vi "Read Network-published IO Shared Variables.vi"() -> (1 "channel errors":errorcluster[](array[cluster]), 2 "data":dbl[](array[numeric]), 3 "UUIDs":string[](array[string])=["Flow Rate [g/s]", "Density [g/cm^3]", "Return Filter dP [psid]", "Outlet Filter and Flowmeter dp [psid]", "Cooler dP [psid]", "Cooler CO2 In [F]", "Cooler CO2 Out [F]", "Pump Frequency [%]", "Recirc Valve Open [%]"])   [LabVIEW 2020]
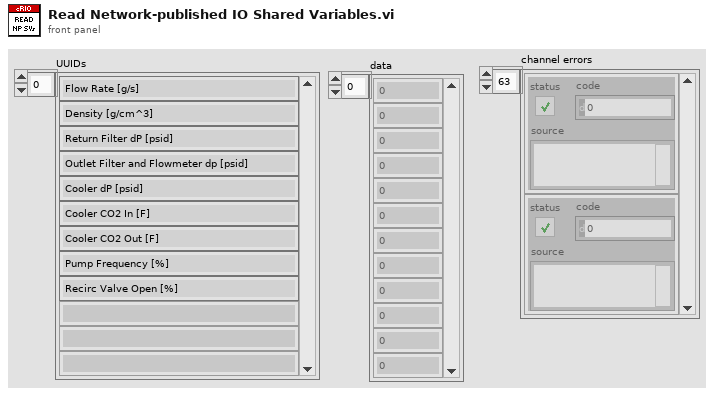
[diagram p1: front panel]
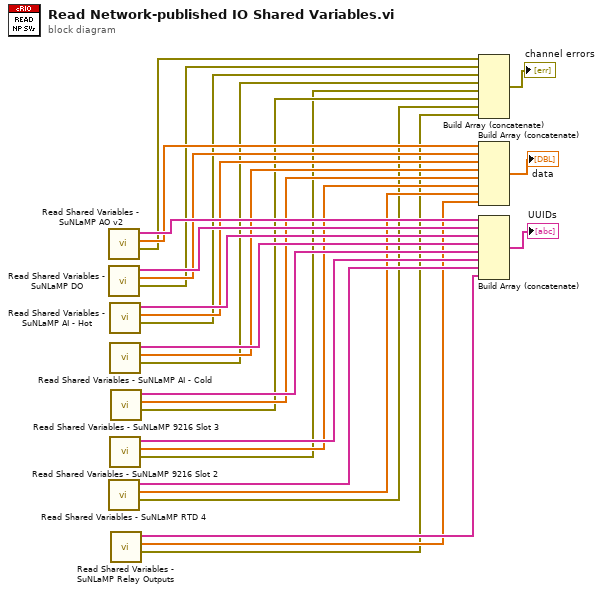
[diagram p0: block diagram]
diagram:
  n1 = call "Read Shared Variables - SuNLaMP AO v2.vi"() -> ("channel errors out"=w16:errorcluster[], "data"=w20:dbl[], "UUIDs"=w27:string[])  [unwired: 9 in]
  n2 = call "Read Shared Variables - SuNLaMP DO.vi"() -> ("channel errors out"=w17:errorcluster[], "data"=w21:dbl[], "UUIDs"=w26:string[])  [unwired: 9 in]
  n3 = call "Read Shared Variables - SuNLaMP RTD 4.vi"() -> ("channel errors out"=w4:errorcluster[], "data"=w5:dbl[], "UUIDs"=w6:string[])  [unwired: 9 in]
  n4 = call "Read Shared Variables - SuNLaMP AI - Hot.vi"() -> ("channel errors out"=w18:errorcluster[], "data"=w22:dbl[], "UUIDs"=w25:string[])  [unwired: 9 in]
  n5 = call "Read Shared Variables - SuNLaMP AI - Cold.vi"() -> ("channel errors out"=w19:errorcluster[], "data"=w23:dbl[], "UUIDs"=w24:string[])  [unwired: 9 in]
  n6 = call "Read Shared Variables - SuNLaMP 9216 Slot 2.vi"() -> ("channel errors out"=w7:errorcluster[], "data"=w8:dbl[], "UUIDs"=w11:string[])  [unwired: 9 in]
  n7 = call "Read Shared Variables - SuNLaMP 9216 Slot 3.vi"() -> ("channel errors out"=w9:errorcluster[], "data"=w10:dbl[], "UUIDs"=w12:string[])  [unwired: 9 in]
  n8 = call "Read Shared Variables - SuNLaMP Relay Outputs.vi"() -> ("channel errors out"=w1:errorcluster[], "data"=w2:dbl[], "UUIDs"=w3:string[])  [unwired: 9 in]
  n9 = Build Array (concatenate)(w16, w17, w18, w19, w7, w9, w4, w1) -> (→"channel errors":errorcluster[])
  n10 = Build Array (concatenate)(w20, w21, w22, w23, w10, w8, w5, w2) -> (→"data":dbl[])
  n11 = Build Array (concatenate)(w27, w26, w25, w24, w12, w11, w6, w3) -> (→"UUIDs":string[])
